vi "Command_Feed.vi"(0 "Startup":bool, 2 "Timeout":dbl) -> (6 "Reint":bool, 7 "Completed":bool, 10 "Output":bool)   [LabVIEW 2020]
uses:
  Auto Utilities/Command_Execution_State.ctl
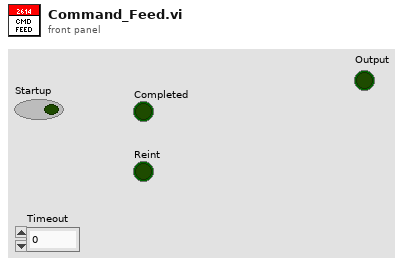
[diagram p1: front panel]
types:
  T1 = typedef "Command_Execution_State.ctl" = enum16{"Initialize", "Execute", "Finish"}
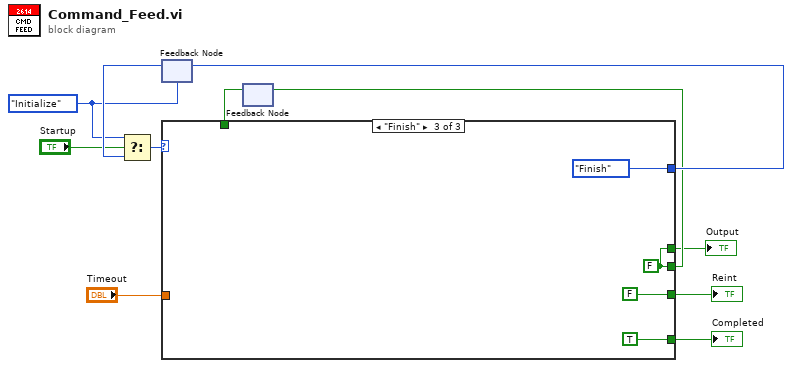
[diagram p0: block diagram]
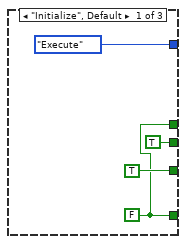
[diagram p2: hidden frame]
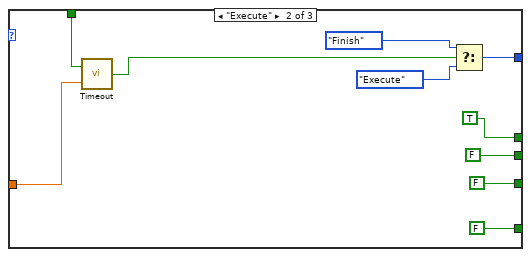
[diagram p3: hidden frame]
diagram:
  w5 = Command_Execution_State."Initialize" ("Play State")
  n1 = feedback #1(w5) -> (w9:T1)
  n2 = Select(t=w5, s="Startup", f=w9) -> (s? t:f=w11:T1)
  n3 = feedback #2() -> (w3:bool)  [unwired: 1 in]
  n4 = case shown="\"Finish\"" w11 {
    tunnel: [Command_Execution_State."Execute" ("Play State") w20 Command_Execution_State."Finish" ("Play State")] -> w10
    tunnel: [w12 FALSE TRUE] -> w8
    tunnel: [TRUE FALSE FALSE] -> w6
    tunnel: [TRUE FALSE w26] -> w4
    tunnel: w3 -> [_ w22 _]
    tunnel: "Timeout" -> [_ w21 _]
    tunnel: [w12 TRUE w26] -> w1
    frame "Initialize", Default {
      w12 = FALSE
    }
    frame "Execute" {
      n5 = call "Timeout.vi"("Timeout"=w21, "Initialize"=w22) -> ("Timed Out?"=w17:bool)
      n6 = Select(t=Command_Execution_State."Finish" ("Play State"), s=w17, f=Command_Execution_State."Execute" ("Play State")) -> (s? t:f=w20:T1)
    }
    frame "Finish" {
      w26 = FALSE
    }
  }
  "Completed" <- w8
  "Reint" <- w6
  "Output" <- w1
  n7 = feedback-in #1(w10) -> ()
  n8 = feedback-in #2(w4) -> ()
